vi "CreateSound.vi"() -> ()   [LabVIEW 2019, in "Initializers.lvlib"]
uses:
  Initializers.lvlib
  <vilib>/sound2/lvsound2.llb/Sound File Read Open.vi
  <vilib>/sound2/lvsound2.llb/Sound File Read (DBL).vi
panel:
  out "Waveform Graph":i16[][](graph)
  out "error out 2":errorcluster
  in  "error out":errorcluster
  in  "Target Path":path=path "C:/Users/FreshBob/Dropbox/VIs/myRIO_GameConsole/Data/Sounds"
  in  "Paths":path=path "C:/Users/FreshBob/Dropbox/VIs/myRIO_GameConsole/Data/Sounds"
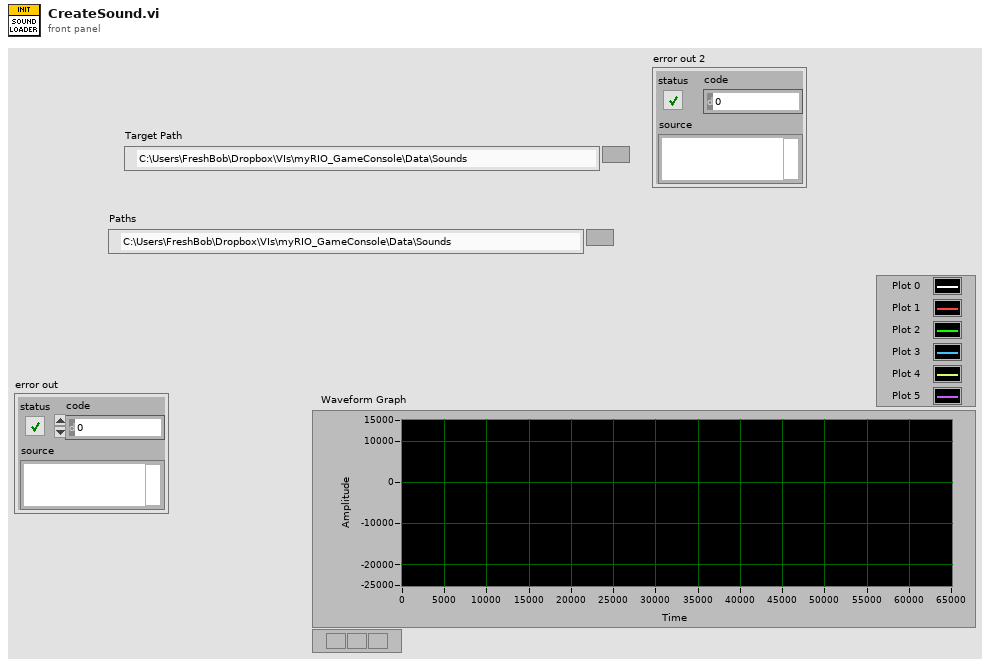
[diagram p1: front panel]
types:
  T1 = enum16{"open", "replace", "create", "open or create", "replace or create", "replace or create with confirmation"}
  T2 = typedef "Sound File Refnum.ctl" = refnum<file>
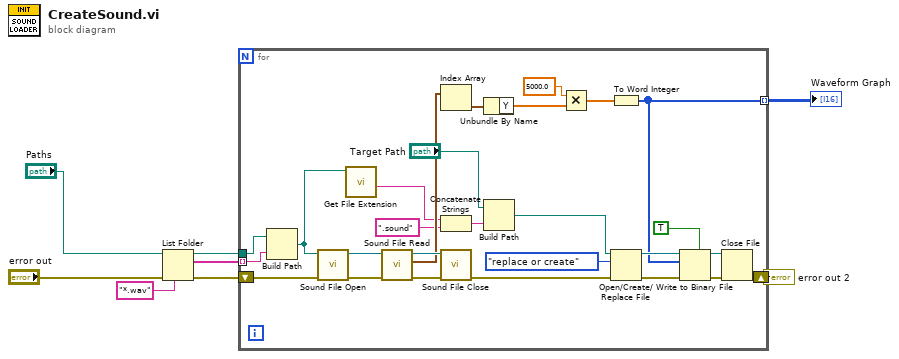
[diagram p0: block diagram]
diagram:
  n1 = List Folder(path="Paths", pattern="*.wav", error in="error out") -> (path out=w4:path, filenames=w1:string[], error out=w6:errorcluster)  [unwired: 1 in, 1 out]
  n2 = for {
    tunnel: w4 -> [w11]
    shift-right: [w27] -> w7
    shift-left: w6 -> [w13]
    tunnel: [w12] -> w2 mode=indexing
    tunnel: w1 -> [w10] mode=indexing
    n3 = Build Path(base path=w11, name or relative path=w10) -> (appended path=w9:path)
    n4 = call-poly <vilib>:"Sound File Open.vi"("error in (no error)"=w13, "path"=w9) -> ("error out"=w24:errorcluster, "sound file refnum"=w25:T2)  [unwired: 8 in]
    n5 = call <vilib>:"Get File Extension.vi"("file"=w9) -> ("filename without extension"=w14:string)  [unwired: 6 in, 4 out]
    n6 = call-poly <vilib>:"Sound File Read.vi"("error in (no error)"=w24, "sound file refnum"=w25) -> ("error out"=w22:errorcluster, "data"=w19:waveform(dbl)[], "sound file refnum out"=w23:T2)  [unwired: 5 in, 2 out]
    n7 = Index Array(array=w19) -> (element=w21:waveform(dbl))  [unwired: 1 in]
    n8 = Concatenate Strings(w14, ".sound" ("string")) -> (w15:string)
    n9 = call <vilib>:"Sound File Close.vi"("error in (no error)"=w22, "sound file refnum"=w23) -> ("error out"=w29:errorcluster)  [unwired: 9 in]
    n10 = Unbundle By Name(w21) -> ("Y"=w20:dbl[])
    n11 = Build Path(base path="Target Path", name or relative path=w15) -> (appended path=w26:path)
    n12 = Multiply(x=5000.0, y=w20) -> (x*y=w18:dbl[])
    n13 = To Word Integer(number=w18) -> (16bit integer=w12:i16[])
    n14 = Open/Create/Replace File(file path (use dialog)=w26, error in=w29, operation (0:open)=T1."replace or create") -> (refnum out=w35:refnum<file>, error out=w34:errorcluster)  [unwired: 3 in, 1 out]
    n15 = Write to Binary File(file (use dialog)=w35, data=w12, error in=w34, 5:TRUE ("prepend array or string size? (T)")) -> (refnum out=w33:refnum<file>, error out=w32:errorcluster)  [unwired: 2 in, 1 out]
    n16 = Close File(refnum=w33, error in=w32) -> (error out=w27:errorcluster)  [unwired: 1 out]
  }
  "error out 2" <- w7
  "Waveform Graph" <- w2
